vi "CLD 4 Event Structure Time Out Front Panel.vi"() -> ()   [LabVIEW 2009]
doc: "CLD 4 exercise"
panel:
  in  "Decrement":bool
  out "Error Out":errorcluster
  in  "Error In":errorcluster
  out "Time Has Elapsed":bool
  out "Count":string
  in  "Increment":bool
  in  "Stop VI":bool
  in  "Timeout Target (s)":dbl
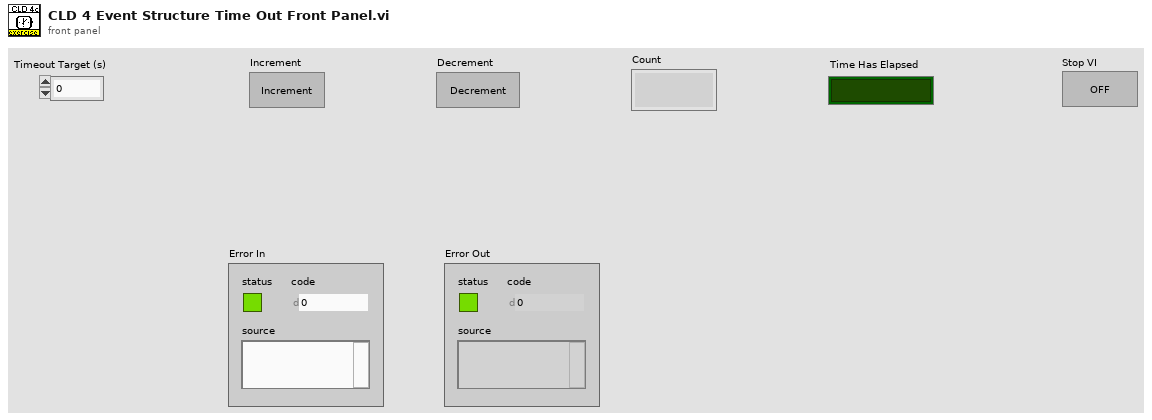
[diagram p1: front panel]
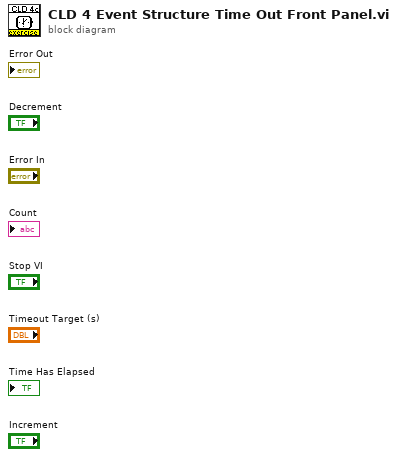
[diagram p0: block diagram]
diagram:
